vi "Main.vi"() -> ()   [LabVIEW 2011]
uses:
  Control 1.ctl
panel:
  in  "05":bool
  in  "04":bool
  in  "03":bool
  out "String":string="Один"
  in  "stop":bool
  in  "02":bool
  in  "01":bool
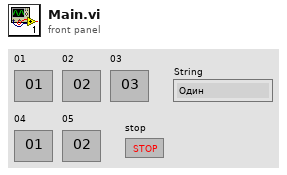
[diagram p1: front panel]
types:
  T1 = typedef "Control 1.ctl" = enum16{"01", "02", "03", "04", "05", "Стоп"}
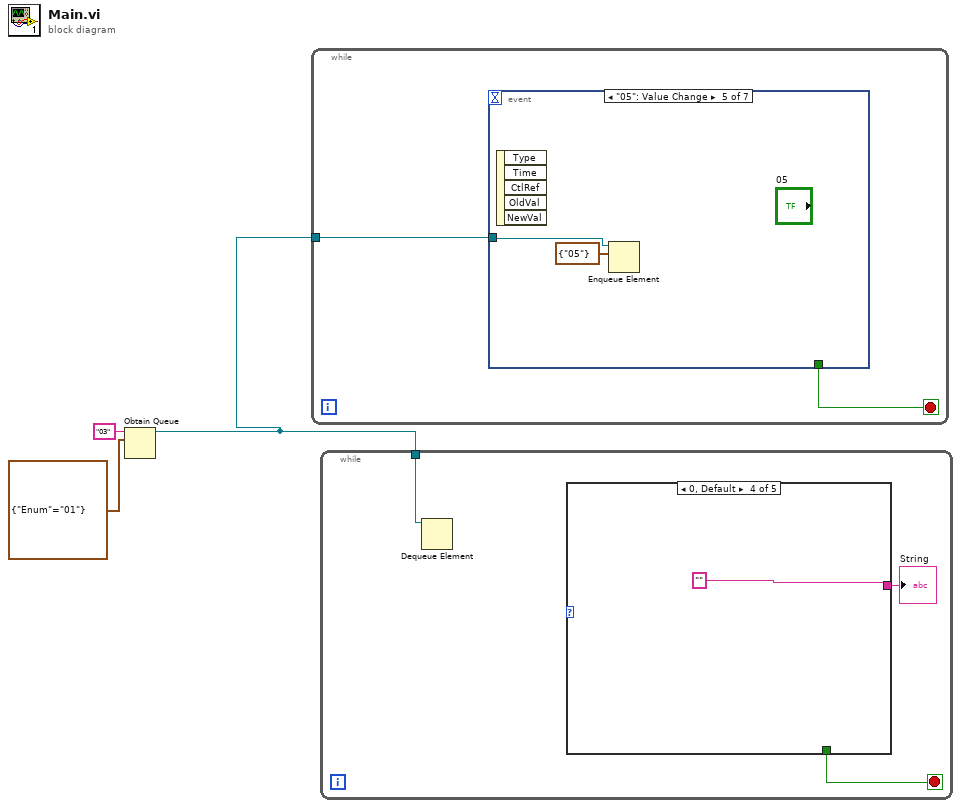
[diagram p0: block diagram]
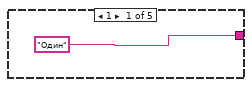
[diagram p2: hidden frame]
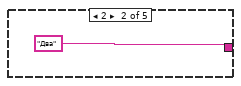
[diagram p3: hidden frame]
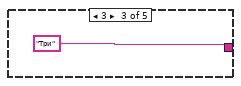
[diagram p4: hidden frame]
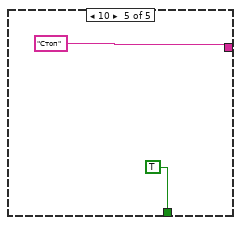
[diagram p5: hidden frame]
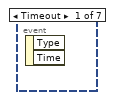
[diagram p6: hidden frame]
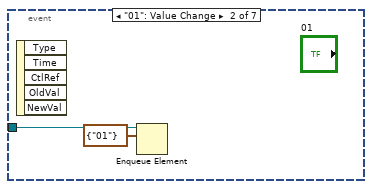
[diagram p7: hidden frame]
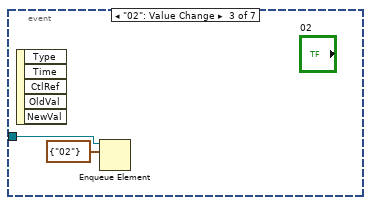
[diagram p8: hidden frame]
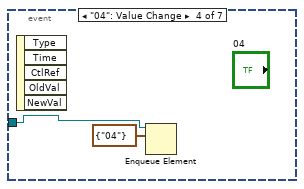
[diagram p9: hidden frame]
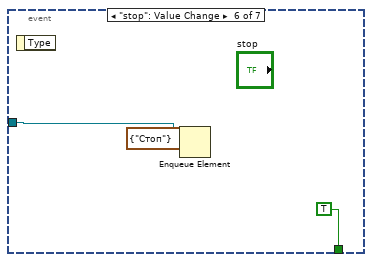
[diagram p10: hidden frame]
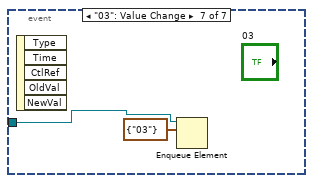
[diagram p11: hidden frame]
diagram:
  n1 = Obtain Queue(name (unnamed)="03", element data type=cluster{"Enum":T1} {"Enum"=enum."01"}) -> (queue out=w2:refnum<queue>)  [unwired: 3 in, 2 out]
  n2 = while {
    tunnel: w2 -> [w5]
    stop <- w4 stop-if-true
    n3 = event shown="[4] \"05\": Value Change" {
      selector: _ -> [_ _ _ _ _ _ _]
      dyn-events: _ -> [_ _ _ _ _ _ _]
      timeout: _ -> [_ _ _ _ _ _ _]
      tunnel: w5 -> [_ w7 w9 w10 w12 w16 w18]
      tunnel: [_ _ _ _ _ TRUE _] -> w4
      event Timeout {
        n4 = event-data() -> ()  [unwired: 1 in, 2 out]
      }
      event "01": Value Change {
        n5 = event-data() -> ()  [unwired: 1 in, 5 out]
        n6 = Enqueue Element(queue=w7, element=cluster{"Enum":T1} {"Enum"=enum."01"}) -> ()  [unwired: 2 in, 3 out]
      }
      event "02": Value Change {
        n7 = event-data() -> ()  [unwired: 1 in, 5 out]
        n8 = Enqueue Element(queue=w9, element=cluster{"Enum":T1} {"Enum"=enum."02"}) -> ()  [unwired: 2 in, 3 out]
      }
      event "04": Value Change {
        n9 = event-data() -> ()  [unwired: 1 in, 5 out]
        n10 = Enqueue Element(queue=w10, element=cluster{"Enum":T1} {"Enum"=enum."04"}) -> ()  [unwired: 2 in, 3 out]
      }
      event "05": Value Change {
        n11 = event-data() -> ()  [unwired: 1 in, 5 out]
        n12 = Enqueue Element(queue=w12, element=cluster{"Enum":T1} {"Enum"=enum."05"}) -> ()  [unwired: 2 in, 3 out]
      }
      event "stop": Value Change {
        n13 = event-data() -> ()  [unwired: 1 in, 1 out]
        n14 = Enqueue Element(queue=w16, element=cluster{"Enum":T1} {"Enum"=enum."Стоп"}) -> ()  [unwired: 2 in, 3 out]
      }
      event "03": Value Change {
        n15 = event-data() -> ()  [unwired: 1 in, 5 out]
        n16 = Enqueue Element(queue=w18, element=cluster{"Enum":T1} {"Enum"=enum."03"}) -> ()  [unwired: 2 in, 3 out]
      }
    }
  }
  n17 = while {
    tunnel: w2 -> [w21]
    stop <- w19 stop-if-true
    n18 = Dequeue Element(queue=w21) -> ()  [unwired: 2 in, 4 out]
    n19 = case shown="0, Default" {
      selector: _ -> [_ _ _ _ _]
      tunnel: ["Один" "Два" "Три" "" "Стоп"] -> w20
      tunnel: [_ _ _ _ TRUE] -> w19
      frame 1 {
      }
      frame 2 {
      }
      frame 3 {
      }
      frame 0, Default {
      }
      frame 10 {
      }
    }
    "String" <- w20
  }
